vi "SHPW Specific Heat of Pure Water (KJ to Kg to K).vi"(1 "Tceg":dbl[unit]) -> (0 "SHPW":dbl[unit])   [LabVIEW 2018]
panel:
  out "Temprature of Pure Water \nKelvin Degree":dbl[unit](slide) scale=273.0..373.0
  out "Tk":dbl[unit]
  out "Temprature of Pure Water\nCentigrade Degree":dbl[unit](slide) scale=0.0..100.0
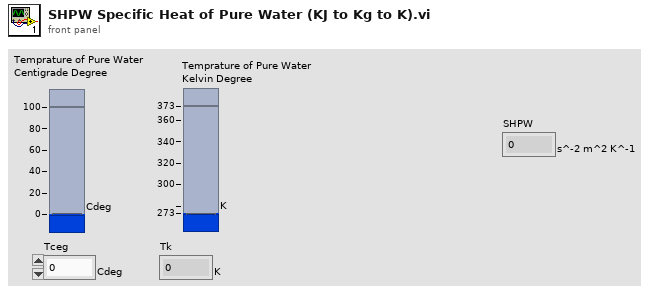
[diagram p1: front panel]
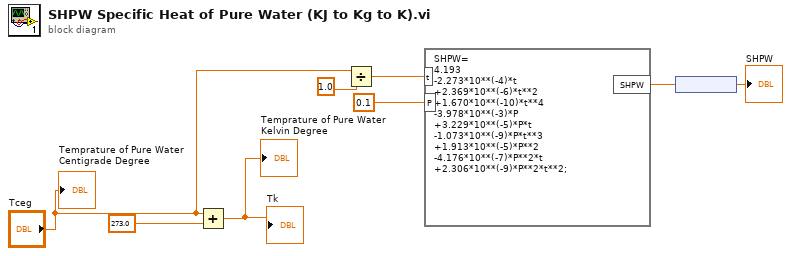
[diagram p0: block diagram]
diagram:
  n1 = Add(x="Tceg", y=dbl[unit] 273.0) -> (x+y=→"Tk" →"Temprature of Pure Water \nKelvin Degree":dbl[unit])
  n2 = Divide(x="Tceg", y=dbl[unit] 1.0) -> (x/y=w8:dbl)
  n3 = formula code="SHPW=\n4.193\n-2.273*10**(-4)*t\n+2.369*10**(-6)*t**2\n+1.670*10**(-10)*t**4\n-3.978*10**(-3)*P\n+3.229*10**(-5)*P*t\n-1.073*10**(-9)*P*t**3\n+1.913*10**(-5)*P**2\n-4.176*10**(-7)*P**2*t\n+2.306*10**(-9)*P**2*t**2;"("t"=w8, "P"=0.1 ("input variable")) -> ("SHPW"=w6:dbl)
  n4 = node(w6) -> (→"SHPW":dbl[unit])
  "Temprature of Pure Water\nCentigrade Degree" <- "Tceg"
